vi "Initialize-link.vi"(8 "error in (no error)":errorcluster, 11 "Motor-GWInstek in":refnum<class "Motor-GWInstek.lvclass">) -> (0 "error out":errorcluster, 3 "Motor-GWInstek out":refnum<class "Motor-GWInstek.lvclass">)   [LabVIEW 2013, in "PowderDeposition.lvlib" / "Motor-GWInstek.lvclass"]
uses:
  Motor-GWInstek.lvclass
  Motor-GWInstek.lvclass/Motor-GWInstek.ctl
  Read Serial Configuration.vi
  <instrlib>/GPD-2303/GPD-2303.lvlib
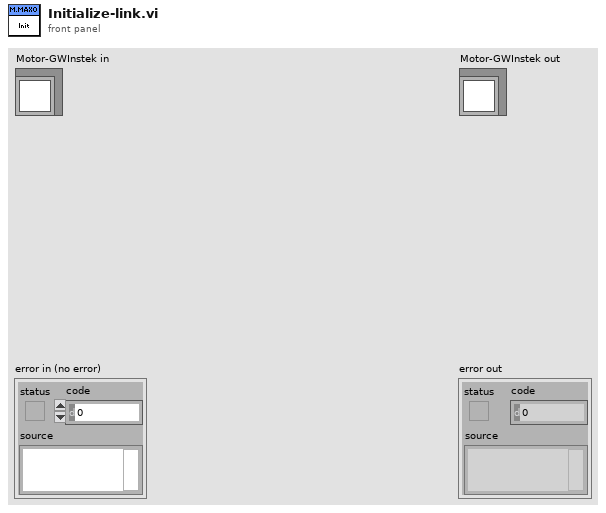
[diagram p1: front panel]
types:
  T1 = cluster{"Baud Rate":u32, "Parity":u16, "Data Bits":u16, "Stop Bits":u16, "Flow Control":u16}
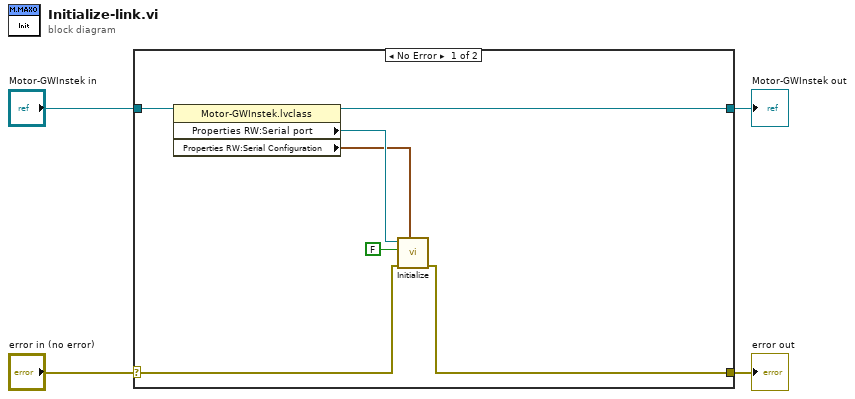
[diagram p0: block diagram]
diagram:
  n1 = case shown="No Error" "error in (no error)" {
    selector: "error in (no error)" -> [w8 w13]
    tunnel: [w9 w13] -> w3
    tunnel: [w5 w12] -> w1
    tunnel: "Motor-GWInstek in" -> [w10 w12]
    frame No Error {
      n2 = property class="Motor-GWInstek.lvclass"(reference=w10) -> (reference out=w5:refnum<class "Motor-GWInstek.lvclass">, "Properties RW:Serial port"=w7:refnum<visa-resource-name>, "Properties RW:Serial Configuration"=w6:T1)  [unwired: 1 in, 1 out]
      n3 = call <instrlib>:"Initialize.vi"("Serial Configuration"=w6, "error in (no error)"=w8, "ID Query (True)"=FALSE, "VISA resource name"=w7) -> ("error out"=w9:errorcluster)  [unwired: 6 in, 1 out]
    }
    frame Error {
    }
  }
  "error out" <- w3
  "Motor-GWInstek out" <- w1
